vi "solar_voy_def Variant Array to Cluster.vi"(7 "Cluster Name":string, 10 "Variant Elements":variant[](array[variant])) -> (2 "Cluster Variant":variant)   [LabVIEW 2018]
doc: "This VI creates a cluster variant from an array of variants."
uses:
  <vilib>/Utility/Data Type/NI_Data Type.lvlib
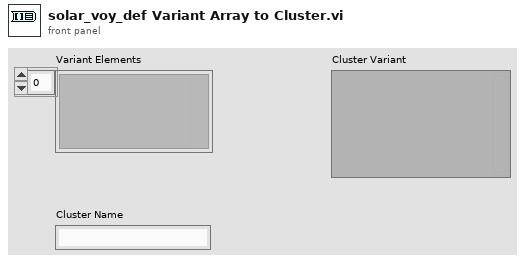
[diagram p1: front panel]
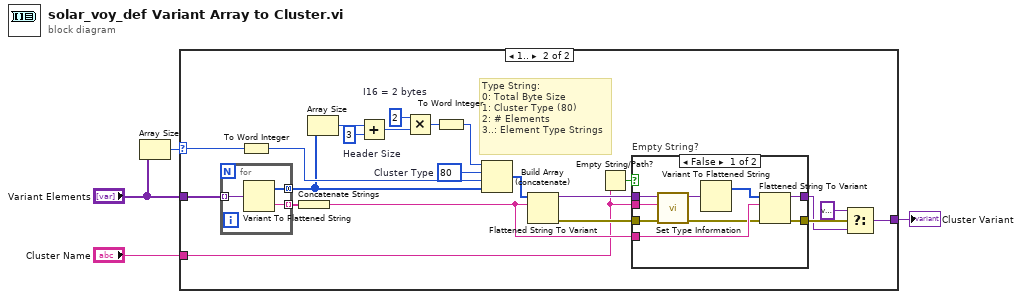
[diagram p0: block diagram]
diagram:
  n1 = Array Size(array="Variant Elements") -> (size(s)=w3:i32)
  n2 = case shown="1.." w3 {
    selector: w3 -> [_ w14]
    tunnel: "Variant Elements" -> [_ w25]
    tunnel: "Cluster Name" -> [_ w10]
    tunnel: [_ w5] -> w1
    frame Default {
      # "Cannot have empty cluster"
    }
    frame 1.. {
      w18 = 2  # I16 = 2 bytes
      w20 = 3  # Header Size
      w22 = i16 80  # Cluster Type
      # "Type String:\n0: Total Byte Size\n1: Cluster Type (80)\n2: # Elements\n3..: Element Type Strings"
      n3 = for {
        tunnel: w25 -> [w40] mode=indexing
        tunnel: [w39] -> w26 mode=indexing
        tunnel: [w38] -> w23 mode=concatenating
        n4 = Variant To Flattened String(Variant=w40) -> (data string=w39:string, 1:w38:i16[])
      }
      n5 = To Word Integer(number=w14) -> (16bit integer=w24:i16)
      n6 = Concatenate Strings(w26) -> (w11:string)
      n7 = Array Size(array=w23) -> (size(s)=w21:i32)
      n8 = Add(x=w21, y=w20) -> (x+y=w19:i32)
      n9 = Multiply(x=w18, y=w19) -> (x*y=w17:i32)
      n10 = To Word Integer(number=w17) -> (16bit integer=w16:i16)
      n11 = Build Array (concatenate)(w16, w22, w24, w23) -> (w15:i16[])
      n12 = Flattened String To Variant(6:w11, 7:w15) -> (0:w12:errorcluster, 3:w13:variant)  [unwired: 1 in]
      n13 = Empty String/Path?(string/path=w10) -> (empty?=w9:bool)
      n14 = case "Empty String?" shown="False" w9 {
        tunnel: w13 -> [w31 w37]
        tunnel: w12 -> [w29 w36]
        tunnel: w11 -> [w34 _]
        tunnel: [w33 w36] -> w7
        tunnel: [w32 w37] -> w6
        tunnel: w10 -> [w30 _]
        frame False {
          n15 = call <vilib>:"Set Type Information.vi"("error in (no error)"=w29, "Name"=w30, "Variant in"=w31) -> ("error out"=w28:errorcluster, "Variant out"=w27:variant)  [unwired: 7 in]
          n16 = Variant To Flattened String(Variant=w27) -> (1:w35:i16[])  [unwired: 1 out]
          n17 = Flattened String To Variant(4:w28, 6:w34, 7:w35) -> (0:w33:errorcluster, 3:w32:variant)
        }
        frame True {
        }
      }
      n18 = Select(t=variant, s=w7, f=w6) -> (s? t:f=w5:variant)
    }
  }
  "Cluster Variant" <- w1
